vi "Add Editor to Core.vi"(8 "error in (no error)":errorcluster, 10 "JKI State Machine Editor Package":path, 11 "JKI State Machine Package":path) -> (0 "error out":errorcluster)   [LabVIEW 2013]
uses:
  <vilib>/Utility/config.llb/Read Key (String).vi
  <vilib>/Utility/config.llb/Write Key (String).vi
  <userlib>/_OpenG.lib/file/file.llb/Valid Path - Traditional__ogtk.vi
  <vilib>/Utility/config.llb/NI_LVConfig.lvlib
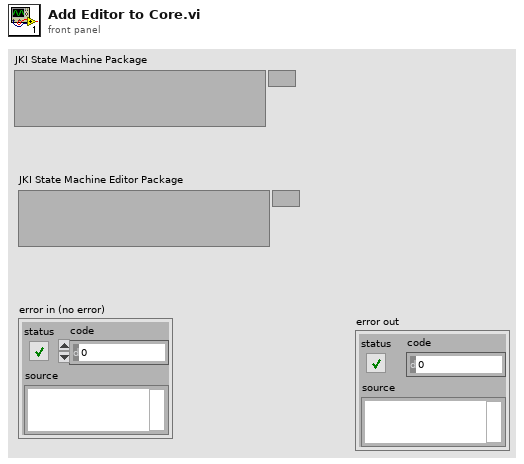
[diagram p1: front panel]
types:
  T1 = cluster{"Num File Groups":i32, "Namespaces":string}
  T2 = typedef "NI_LVConfig.lvlib/Config Data RefNum.ctl" = refnum<k1>
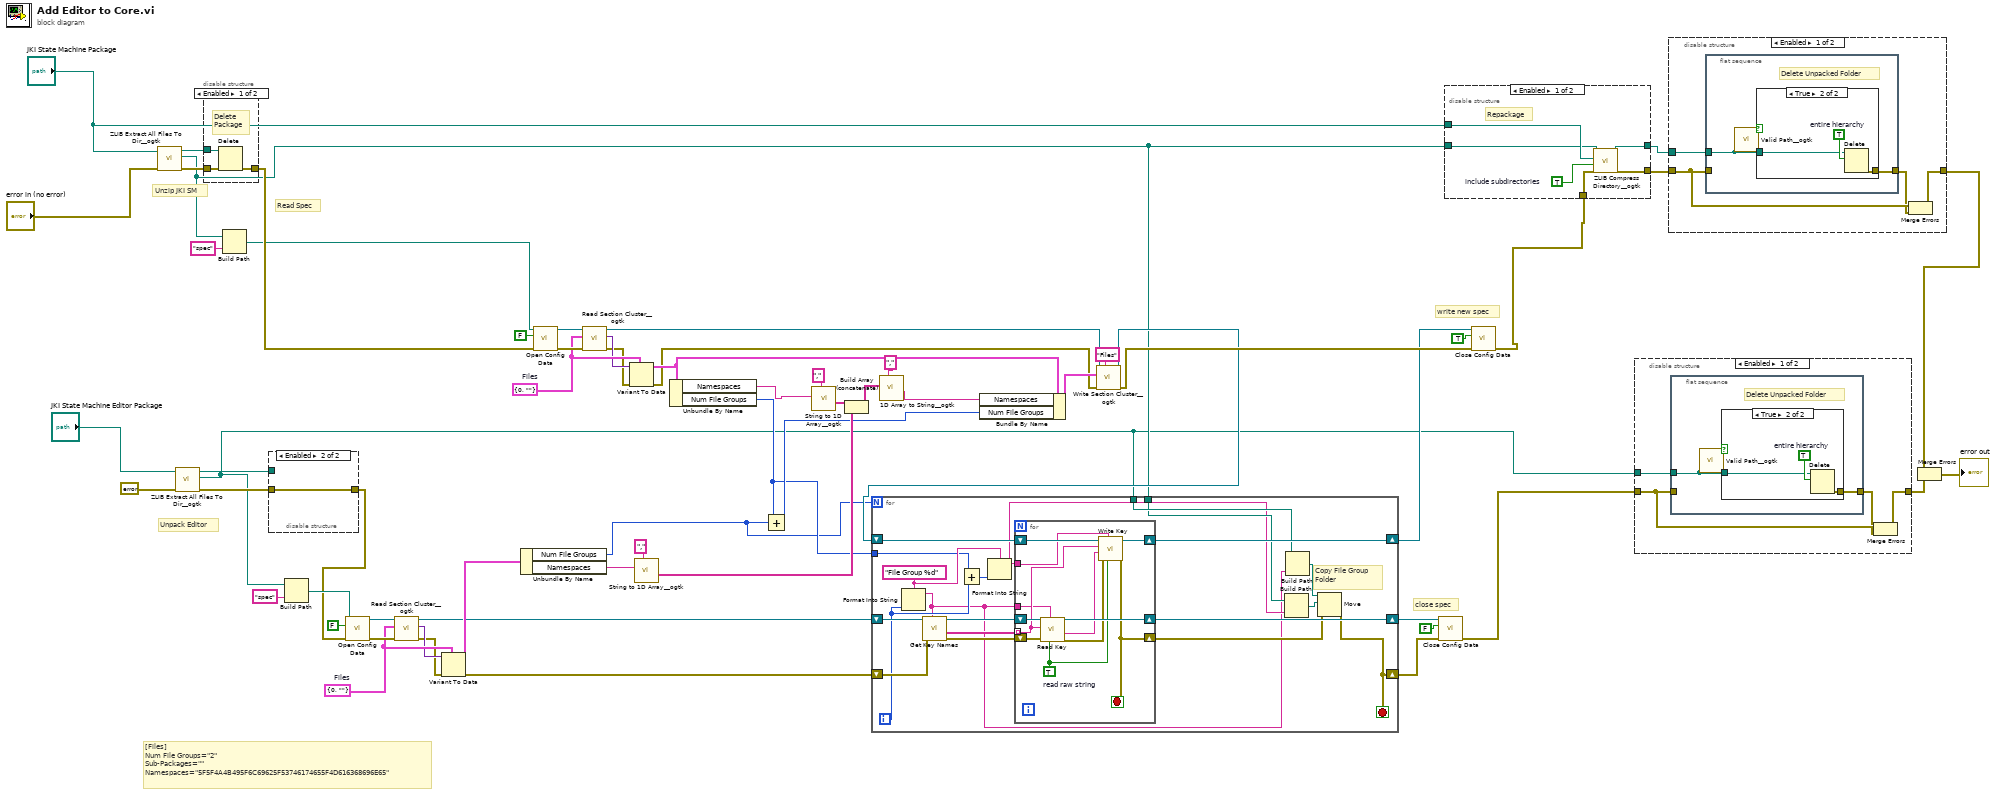
[diagram p0: block diagram]
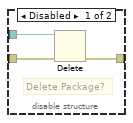
[diagram p8: hidden frame]
diagram:
  w39 = T1 {"Num File Groups"=0, "Namespaces"=""}  # Files
  w46 = T1 {"Num File Groups"=0, "Namespaces"=""}  # Files
  # "close spec"
  # "write new spec"
  # "[Files]\nNum File Groups=\"2\"\nSub-Packages=\"\"\nNamespaces=\"5F5F4A4B495F6C69625F53746174655F4D616368696E65\""
  # "Read Spec"
  # "Unzip JKI SM"
  # "Unpack Editor"
  n1 = call <userlib>:"ZLIB Extract All Files To Dir__ogtk.vi"("error in (no error)"="error in (no error)", "archive name (file dialog)"="JKI State Machine Package") -> ("error out"=w56:errorcluster, "root directory out"=w5:path, "archive name out"=w57:path)  [unwired: 7 in]
  n2 = call <userlib>:"ZLIB Extract All Files To Dir__ogtk.vi"("error in (no error)"=errorcluster {"status"=FALSE, "code"=0, "source"=""}, "archive name (file dialog)"="JKI State Machine Editor Package") -> ("error out"=w55:errorcluster, "root directory out"=w4:path, "archive name out"=w54:path)  [unwired: 7 in]
  n3 = disable-structure shown="Enabled" {
    disable-tunnel: [w65 w66] -> w59
    disable-tunnel: w57 -> [w64 _]
    disable-tunnel: w56 -> [w63 w66]
    frame Enabled {
      # "Delete\nPackage"
      n4 = Delete(path (use dialog)=w64, error in=w63) -> (error out=w65:errorcluster)  [unwired: 3 in, 2 out]
    }
    frame Disabled {
    }
  }
  n5 = Build Path(base path=w5, name or relative path="spec") -> (appended path=w35:path)
  n6 = disable-structure shown="Enabled" {
    disable-tunnel: w55 -> [w69 w70]
    disable-tunnel: w54 -> [w68 _]
    disable-tunnel: [w67 w70] -> w34
    frame Disabled {
      # "Delete Package?"
      n7 = Delete(path (use dialog)=w68, error in=w69) -> (error out=w67:errorcluster)  [unwired: 3 in, 2 out]
    }
    frame Enabled {
    }
  }
  n8 = Build Path(base path=w4, name or relative path="spec") -> (appended path=w50:path)
  n9 = call <vilib>:"Open Config Data.vi"("error in (no error)"=w34, "create file if necessary (T)"=FALSE, "configuration file path"=w50) -> ("error out"=w47:errorcluster, "refnum"=w48:T2)  [unwired: 6 in, 1 out]
  n10 = call <userlib>:"Read Section Cluster__ogtk.vi"("error in (no error)"=w47, "Section Formatted Cluster Type"=w46, "refnum"=w48) -> ("error out"=w44:errorcluster, "Section Formatted Cluster"=w45:variant, "dup refnum"=w14:T2)  [unwired: 4 in, 2 out]
  n11 = Variant To Data(error in=w44, type=w46, Variant=w45) -> (data=w33:T1, error out=w16:errorcluster)
  n12 = Unbundle By Name(w33) -> ("Num File Groups"=w9:i32, "Namespaces"=w32:string)
  n13 = call <vilib>:"Open Config Data.vi"("error in (no error)"=w59, "create file if necessary (T)"=FALSE, "configuration file path"=w35) -> ("error out"=w40:errorcluster, "refnum"=w41:T2)  [unwired: 6 in, 1 out]
  n14 = call <userlib>:"Read Section Cluster__ogtk.vi"("error in (no error)"=w40, "Section Formatted Cluster Type"=w39, "refnum"=w41) -> ("error out"=w37:errorcluster, "Section Formatted Cluster"=w38:variant, "dup refnum"=w17:T2)  [unwired: 4 in, 2 out]
  n15 = Variant To Data(error in=w37, type=w39, Variant=w38) -> (data=w26:T1, error out=w19:errorcluster)
  n16 = call <userlib>:"String to 1D Array__ogtk.vi"("delimiter (Tab)"=",", "string"=w32) -> ("Array of Strings"=w27:string[])  [unwired: 9 in]
  n17 = Unbundle By Name(w26) -> ("Namespaces"=w29:string, "Num File Groups"=w12:i32)
  n18 = Add(x=w12, y=w9) -> (x+y=w25:i32)
  n19 = call <userlib>:"String to 1D Array__ogtk.vi"("delimiter (Tab)"=",", "string"=w29) -> ("Array of Strings"=w28:string[])  [unwired: 9 in]
  n20 = Build Array (concatenate)(w28, w27) -> (w24:string[])
  n21 = call <userlib>:"1D Array to String__ogtk.vi"("delimiter (Tab)"=",", "Array of Strings"=w24) -> ("delimited string"=w22:string)  [unwired: 9 in]
  n22 = Bundle By Name(cluster=w26, "Namespaces"=w22, "Num File Groups"=w25) -> (w21:T1)
  n23 = call <userlib>:"Write Section Cluster__ogtk.vi"("section (optional)"="Files", "error in (no error)"=w19, "Section Formatted Cluster"=w21, "refnum"=w17) -> ("error out"=w18:errorcluster, "dup refnum"=w11:T2)  [unwired: 6 in]
  n24 = for {
    N: w9 -> [_]
    shift-right: [w87] -> w13
    shift-left: w14 -> [w89]
    shift-right: [w77] -> w15
    shift-left: w16 -> [w90]
    shift-right: [w79] -> w10
    shift-left: w11 -> [w84]
    tunnel: w12 -> [w81]
    tunnel: w5 -> [w73]
    tunnel: w4 -> [w74]
    i -> [w80]
    stop <- w77 stop-if-true
    w83 = "File Group %d" ("section")
    # "Copy File Group\nFolder"
    n25 = Format Into String(format string=w83, w80) -> (resulting string=w71:string)  [unwired: 2 in, 1 out]
    n26 = call <vilib>:"Get Key Names.vi"("section"=w71, "error in (no error)"=w90, "refnum"=w89) -> ("error out"=w86:errorcluster, "key names"=w85:string[], "refnum out"=w88:T2)  [unwired: 5 in, 1 out]
    n27 = Add(x=w81, y=w80) -> (x+y=w82:i32)
    n28 = Format Into String(format string=w83, w82) -> (resulting string=w72:string)  [unwired: 2 in, 1 out]
    n29 = for {
      tunnel: w71 -> [w93]
      shift-right: [w91] -> w78
      shift-left: w86 -> [w100]
      shift-right: [w101] -> w87
      shift-left: w88 -> [w102]
      tunnel: w85 -> [w95] mode=indexing
      shift-right: [w96] -> w79
      shift-left: w84 -> [w99]
      tunnel: w72 -> [w92]
      stop <- w91 stop-if-true
      w98 = TRUE  # read raw string
      n30 = call-poly <vilib>:"Read Key.vi"("read raw string? (F)"=w98, "section"=w93, "error in (no error)"=w100, "key"=w95, "refnum"=w102) -> ("error out"=w97:errorcluster, "value"=w94:string, "refnum out"=w101:T2)  [unwired: 3 in, 1 out]
      n31 = call-poly <vilib>:"Write Key.vi"("write raw string? (F)"=w98, "section"=w92, "error in (no error)"=w97, "value"=w94, "key"=w95, "refnum"=w99) -> ("error out"=w91:errorcluster, "refnum out"=w96:T2)  [unwired: 3 in, 1 out]
    }
    n32 = Build Path(base path=w73, name or relative path=w72) -> (appended path=w76:path)
    n33 = Build Path(base path=w74, name or relative path=w71) -> (appended path=w75:path)
    n34 = Move(source path=w75, error in=w78, 10:w76) -> (error out=w77:errorcluster)  [unwired: 2 in, 2 out]
  }
  n35 = call <vilib>:"Close Config Data.vi"("error in (no error)"=w15, "write file if changed (T)"=FALSE, "refnum"=w13) -> ("error out"=w8:errorcluster)  [unwired: 7 in, 1 out]
  n36 = call <vilib>:"Close Config Data.vi"("error in (no error)"=w18, "write file if changed (T)"=TRUE, "refnum"=w10) -> ("error out"=w58:errorcluster)  [unwired: 7 in, 1 out]
  n37 = disable-structure shown="Enabled" {
    disable-tunnel: "JKI State Machine Package" -> [w108 _]
    disable-tunnel: [w107 w109] -> w3
    disable-tunnel: [w106 w110] -> w2
    disable-tunnel: w58 -> [w105 w109]
    disable-tunnel: w5 -> [w103 w110]
    frame Enabled {
      w104 = TRUE  # include subdirectories
      # "Repackage"
      n38 = call <userlib>:"ZLIB Compress Directory__ogtk.vi"("error in (no error)"=w105, "include subdirectories (F)"=w104, "archive name (root directory with .zip ending)"=w108, "root directory (file dialog)"=w103) -> ("error out"=w107:errorcluster, "root directory out"=w106:path)  [unwired: 5 in, 1 out]
    }
    frame Disabled {
    }
  }
  n39 = disable-structure shown="Enabled" {
    disable-tunnel: w4 -> [w114 _]
    disable-tunnel: w8 -> [w113 _]
    disable-tunnel: [w111 _] -> w7
    frame Enabled {
      n40 = flat-sequence {
        tunnel: w114 -> [w116]
        tunnel: w113 -> [_]
        tunnel: [w117] -> w112
        frame #0 {
          # "Delete Unpacked Folder"
          n41 = call-poly <userlib>:"Valid Path__ogtk.vi"("path"=w116) -> ("valid"=w115:bool)
          n42 = case shown="True" w115 {
            tunnel: [_ w119] -> w117
            tunnel: w116 -> [_ w118]
            frame False {
            }
            frame True {
              w120 = TRUE  # entire hierarchy
              n43 = Delete(path (use dialog)=w118, entire hierarchy (F)=w120) -> (error out=w119:errorcluster)  [unwired: 3 in, 2 out]
            }
          }
        }
      }
      n44 = Merge Errors(w113, w112) -> (w111:errorcluster)
    }
    frame Disabled {
    }
  }
  n45 = disable-structure shown="Enabled" {
    disable-tunnel: w2 -> [w124 _]
    disable-tunnel: w3 -> [w123 _]
    disable-tunnel: [w121 _] -> w1
    frame Enabled {
      n46 = flat-sequence {
        tunnel: w124 -> [w126]
        tunnel: w123 -> [_]
        tunnel: [w127] -> w122
        frame #0 {
          # "Delete Unpacked Folder"
          n47 = call-poly <userlib>:"Valid Path__ogtk.vi"("path"=w126) -> ("valid"=w125:bool)
          n48 = case shown="True" w125 {
            tunnel: [_ w129] -> w127
            tunnel: w126 -> [_ w128]
            frame False {
            }
            frame True {
              w130 = TRUE  # entire hierarchy
              n49 = Delete(path (use dialog)=w128, entire hierarchy (F)=w130) -> (error out=w129:errorcluster)  [unwired: 3 in, 2 out]
            }
          }
        }
      }
      n50 = Merge Errors(w123, w122) -> (w121:errorcluster)
    }
    frame Disabled {
    }
  }
  n51 = Merge Errors(w1, w7) -> (→"error out":errorcluster)
